vi "l_model_backward.vi"(1 "caches":T1(array[cluster]), 2 "Y":dbl[][](array[numeric]), 3 "AL":dbl[][](array[numeric])) -> (0 "grads":map{string, dbl[][]}(c390))   [LabVIEW 2020]
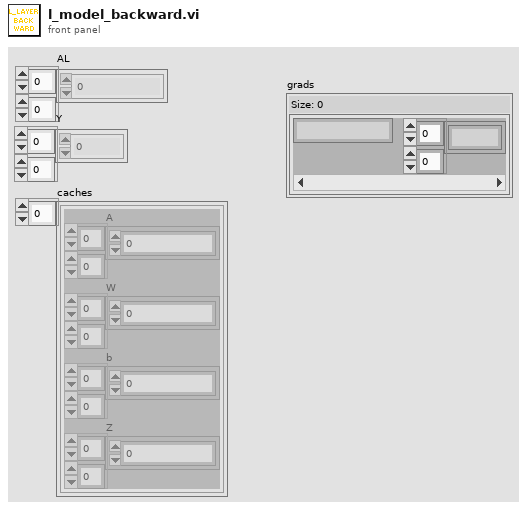
[diagram p1: front panel]
types:
  T1 = cluster{"A":dbl[][], "W":dbl[][], "b":dbl[][], "Z":dbl[][]}[]
  T2 = cluster{"A":dbl[][], "W":dbl[][], "b":dbl[][], "Z":dbl[][]}
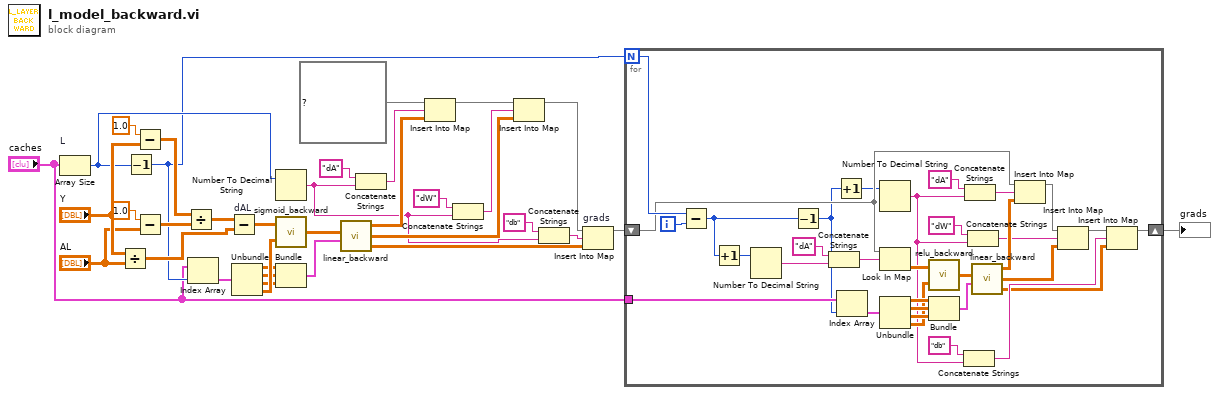
[diagram p0: block diagram]
diagram:
  n1 = Array Size "L"(array="caches") -> (size(s)=w15:i32)
  n2 = Divide(x="Y", y="AL") -> (x/y=w28:dbl[][])
  n3 = Decrement(x=w15) -> (x-1=w4:i32)
  n4 = Subtract(x=1.0, y="Y") -> (x-y=w32:dbl[][])
  n5 = Subtract(x=1.0, y="AL") -> (x-y=w29:dbl[][])
  n6 = Divide(x=w32, y=w29) -> (x/y=w27:dbl[][])
  n7 = Index Array(array="caches", index=w4) -> (element=w26:T2)
  n8 = Subtract "dAL"(x=w27, y=w28) -> (x-y=w24:dbl[][])
  n9 = Unbundle(w26) -> ("A"=w22:dbl[][], "W"=w21:dbl[][], "b"=w20:dbl[][], "Z"=w25:dbl[][])
  n10 = Number To Decimal String(number=w15) -> (decimal integer string=w6:string)  [unwired: 1 in]
  n11 = call "sigmoid_backward.vi"("Z"=w25, "dA"=w24) -> ("dZ"=w23:dbl[][])
  n12 = Bundle("A"=w22, "W"=w21, "b"=w20) -> (w19:cluster{"A":dbl[][], "W":dbl[][], "b":dbl[][]})  [unwired: 1 in]
  n13 = call "linear_backward.vi"("cache"=w19, "dZ"=w23) -> ("db"=w8:dbl[][], "dW"=w12:dbl[][], "dA_prev"=w14:dbl[][])  [unwired: 2 in]
  n14 = Concatenate Strings("dA" ("string"), w6) -> (w17:string)
  n15 = Insert Into Map(map in=map{string, dbl[][]} {} ("Map"), key=w17, value=w14) -> (map out=w13:map{string, dbl[][]})  [unwired: 2 out]
  n16 = Concatenate Strings("dW" ("string"), w6) -> (w11:string)
  n17 = Insert Into Map(map in=w13, key=w11, value=w12) -> (map out=w9:map{string, dbl[][]})  [unwired: 2 out]
  n18 = Concatenate Strings("db" ("string"), w6) -> (w7:string)
  n19 = Insert Into Map "grads"(map in=w9, key=w7, value=w8) -> (map out=w2:map{string, dbl[][]})  [unwired: 2 out]
  n20 = for {
    N: w4 -> [w66]
    tunnel: "caches" -> [w64]
    shift-right: [w36] -> w1
    shift-left: w2 -> [w51]
    i -> [w65]
    n21 = Subtract(x=w66, y=w65) -> (x-y=w54:i32)
    n22 = Increment(x=w54) -> (x+1=w35:i32)
    n23 = Number To Decimal String(number=w35) -> (decimal integer string=w55:string)  [unwired: 1 in]
    n24 = Decrement(x=w54) -> (x-1=w48:i32)
    n25 = Concatenate Strings("dA" ("string"), w55) -> (w56:string)
    n26 = Increment(x=w48) -> (x+1=w47:i32)
    n27 = Index Array(array=w64, index=w48) -> (element=w63:T2)
    n28 = Number To Decimal String(number=w47) -> (decimal integer string=w39:string)  [unwired: 1 in]
    n29 = Look In Map(map=w51, key=w56) -> (value=w52:dbl[][])  [unwired: 1 in, 1 out]
    n30 = Unbundle(w63) -> ("A"=w60:dbl[][], "W"=w59:dbl[][], "b"=w58:dbl[][], "Z"=w57:dbl[][])
    n31 = call "relu_backward.vi"("Z"=w57, "dA"=w52) -> ("dZ"=w62:dbl[][])
    n32 = Bundle("A"=w60, "W"=w59, "b"=w58) -> (w61:cluster{"A":dbl[][], "W":dbl[][], "b":dbl[][]})  [unwired: 1 in]
    n33 = Concatenate Strings("db" ("string"), w39) -> (w40:string)
    n34 = Concatenate Strings("dA" ("string"), w39) -> (w50:string)
    n35 = Concatenate Strings("dW" ("string"), w39) -> (w44:string)
    n36 = call "linear_backward.vi"("cache"=w61, "dZ"=w62) -> ("db"=w37:dbl[][], "dW"=w42:dbl[][], "dA_prev"=w46:dbl[][])  [unwired: 2 in]
    n37 = Insert Into Map(map in=w51, key=w50, value=w46) -> (map out=w45:map{string, dbl[][]})  [unwired: 2 out]
    n38 = Insert Into Map(map in=w45, key=w44, value=w42) -> (map out=w41:map{string, dbl[][]})  [unwired: 2 out]
    n39 = Insert Into Map(map in=w41, key=w40, value=w37) -> (map out=w36:map{string, dbl[][]})  [unwired: 2 out]
  }
  "grads" <- w1
